vi "Intake_Motor_global.vi"() -> ()   [LabVIEW 2020]
uses:
  Subsystems/Intake/Intake_cluster.ctl
  Subsystems/Intake/Intake_control_states.ctl
  <vilib>/Rock Robotics/WPI/Solenoid/WPI_SolenoidValue.ctl
panel:
  in  "Intake_pneumatic^2":T1=enum."Reverse"
  in  "Intake_motor^2":dbl
  in  "Intake_pnuematic":string="Intake_pnuematic"
  in  "Intake_Execute_Notifier":refnum<notifier>
  in  "Intake_set_notifier":refnum<notifier>
  in  "Intake_set_ref":string="Intake_set_ref"
  in  "Intake_execute_ref":string="Intake_execute_ref"
  in  "Intake_motor":string="Intake_motor"
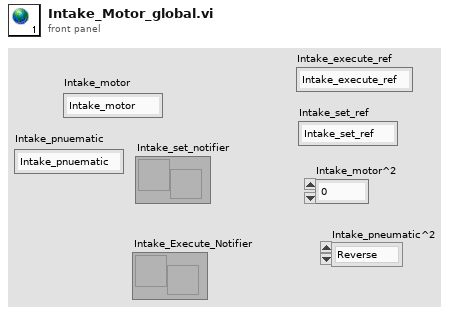
[diagram p1: front panel]
types:
  T1 = typedef "WPI_SolenoidValue.ctl" = enum16{"Off", "On", "Forward", "Reverse"}
diagram:
